vi "thermo_K_conver.vi"(8 "y":dbl=1000000.0, 10 "Measurement Data[1]":dbl, 11 "Measurement Data[0]":dbl) -> (3 "Result":dbl)   [LabVIEW 2011]
uses:
  <vilib>/express/express arith-compare/Formula/XNode/ExpressFormulaBlockNode.xnode
  <vilib>/ptbypt/NI_PtbyPt.lvlib
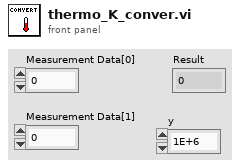
[diagram p1: front panel]
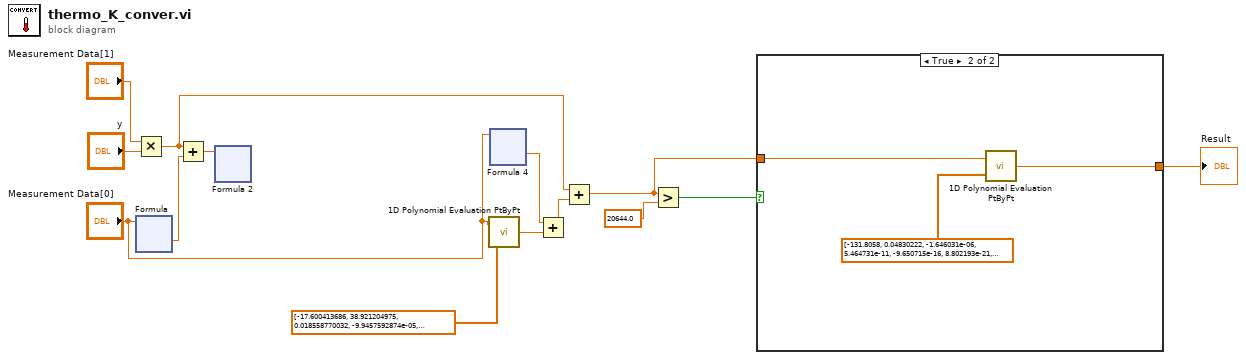
[diagram p0: block diagram]
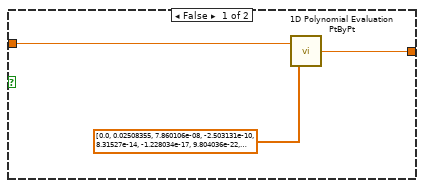
[diagram p2: hidden frame]
diagram:
  n1 = Multiply(x="Measurement Data[1]", y="y") -> (x*y=w2:dbl)
  n2 = xnode ("Formula")("T"="Measurement Data[0]") -> ("Result"=w11:dbl)  [unwired: 1 in, 1 out]
  n3 = Add(x=w2, y=w11) -> (x+y=w12:dbl)
  n4 = xnode ("Formula 2")("V"=w12) -> ()  [unwired: 1 in, 2 out]
  n5 = call <vilib>:"1D Polynomial Evaluation PtByPt.vi"("Coefficients: a"=dbl[] [-17.600413686, 38.921204975, 0.018558770032, -9.9457592874e-05, 3.1840945719e-07, -5.6072844889e-10, 5.6075059059e-13, -3.2020720003e-16, 9.7151147152e-20, -1.2104721275e-23], "x"="Measurement Data[0]") -> ("y"=w9:dbl)
  n6 = xnode ("Formula 4")("T"="Measurement Data[0]") -> ("Result"=w8:dbl)  [unwired: 1 in, 1 out]
  n7 = Add(x=w8, y=w9) -> (x+y=w3:dbl)
  n8 = Add(x=w2, y=w3) -> (x+y=w1:dbl)
  n9 = Greater?(x=w1, y=20644.0) -> (0:w5:bool)
  n10 = case shown="True" w5 {
    tunnel: w1 -> [w15 w19]
    tunnel: [w16 w18] -> w4
    frame False {
      n11 = call <vilib>:"1D Polynomial Evaluation PtByPt.vi"("Coefficients: a"=dbl[] [0.0, 0.02508355, 7.860106e-08, -2.503131e-10, 8.31527e-14, -1.228034e-17, 9.804036e-22, -4.41303e-26, 1.057734e-30, -1.052755e-35], "x"=w15) -> ("y"=w16:dbl)
    }
    frame True {
      n12 = call <vilib>:"1D Polynomial Evaluation PtByPt.vi"("Coefficients: a"=dbl[] [-131.8058, 0.04830222, -1.646031e-06, 5.464731e-11, -9.650715e-16, 8.802193e-21, -3.11081e-26], "x"=w19) -> ("y"=w18:dbl)
    }
  }
  "Result" <- w4
